vi "波形图标（显示两个测量结果的实时波形）.vi"() -> ()   [LabVIEW 2017]
panel:
  out "波形图表 2":T1(graph)
  in  "布尔 2":bool
  in  "布尔":bool
  out "波形图表":T1(graph)
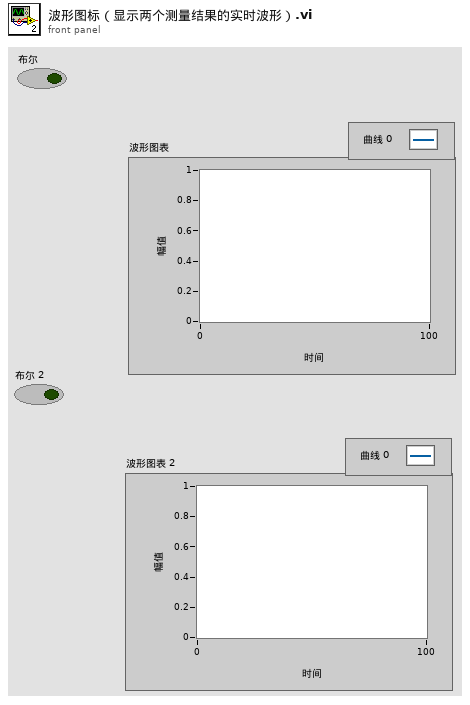
[diagram p1: front panel]
types:
  T1 = cluster{"number: 0 to 1":dbl, "number: 0 to 1":dbl}
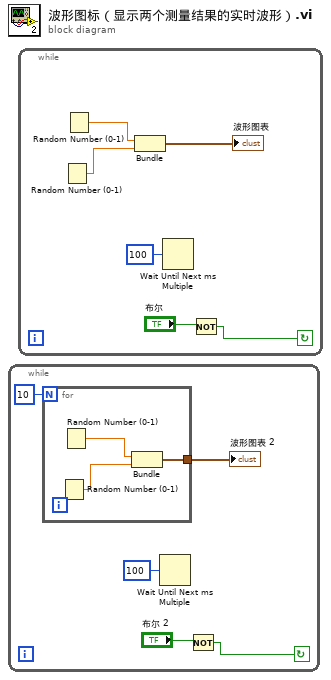
[diagram p0: block diagram]
diagram:
  n1 = while {
    stop <- w2 continue-if-true
    n2 = for {
      N: 10 -> [_]
      tunnel: [w6] -> w5
      n3 = Random Number (0-1)() -> (number: 0 to 1=w7:dbl)
      n4 = Random Number (0-1)() -> (number: 0 to 1=w8:dbl)
      n5 = Bundle("number: 0 to 1"=w8, "number: 0 to 1"=w7) -> (w6:T1)  [unwired: 1 in]
    }
    "波形图表 2" <- w5
    n6 = Wait Until Next ms Multiple(millisecond multiple=u32 100 ("毫秒倍数")) -> ()  [unwired: 1 out]
    n7 = Not(x="布尔 2") -> (.not. x?=w2:bool)
  }
  n8 = while {
    stop <- w9 continue-if-true
    n9 = Random Number (0-1)() -> (number: 0 to 1=w13:dbl)
    n10 = Random Number (0-1)() -> (number: 0 to 1=w14:dbl)
    n11 = Bundle("number: 0 to 1"=w14, "number: 0 to 1"=w13) -> (→"波形图表":T1)  [unwired: 1 in]
    n12 = Wait Until Next ms Multiple(millisecond multiple=u32 100 ("毫秒倍数")) -> ()  [unwired: 1 out]
    n13 = Not(x="布尔") -> (.not. x?=w9:bool)
  }
